vi "PFI-28000-Channel_Set Test Mode.vi"(8 "error in (no error)":errorcluster, 10 "Test Mode":string, 11 "PFI-28000-Channel in":refnum<class "PFI-28000-Channel.lvclass">) -> (0 "error out":errorcluster, 3 "PFI-28000-Channel out":refnum<class "PFI-28000-Channel.lvclass">)   [LabVIEW 2017, in "PFI-28000-Channel.lvclass"]
uses:
  PFI-28000-Channel.lvclass
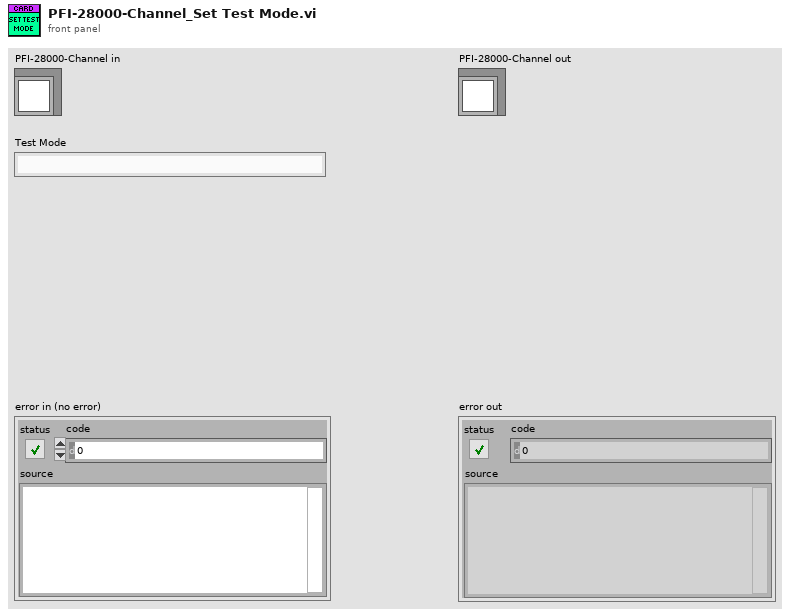
[diagram p1: front panel]
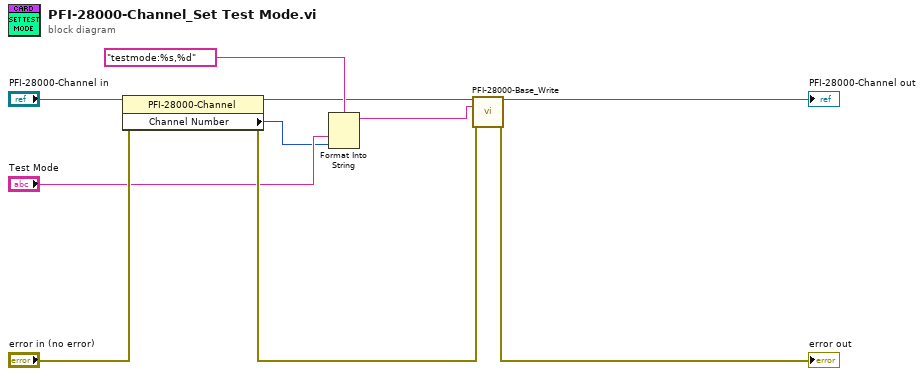
[diagram p0: block diagram]
diagram:
  n1 = property class="PFI-28000-Channel"(reference="PFI-28000-Channel in", error in="error in (no error)") -> (reference out=w6:refnum<class "PFI-28000-Channel.lvclass">, error out=w4:errorcluster, "Channel Number"=w1:i32)
  n2 = Format Into String(format string="testmode:%s,%d" ("empty string"), "Test Mode", w1) -> (resulting string=w3:string)  [unwired: 2 in, 1 out]
  n3 = call-dynamic "PFI-28000-Base_Write.vi"("PFI-28000-Base in"=w6, "Command"=w3, "error in (no error)"=w4) -> ("PFI-28000-Base out"=→"PFI-28000-Channel out":refnum<class "PFI-28000-Channel.lvclass">, "error out"=→"error out":errorcluster)  [unwired: 11 in]
